vi "82_Ultrasonic_map.vi"() -> ()   [LabVIEW 2018]
uses:
  <userlib>/KNR OS 4.0 LabVIEW Toolkit/Type Definition/Resource.ctl
  <userlib>/KNR OS 3.0 LabVIEW Toolkit/Type Definition/Ultrasonic Port Number.ctl
  <userlib>/KNR OS 4.0 LabVIEW Toolkit/Type Definition/RC Servo Port.ctl
panel:
  out "Dist 1(cm)":dbl
  out "XY Graph":cluster{dbl[], dbl[]}(graph)
  in  "stop":bool
  # "500~2500"
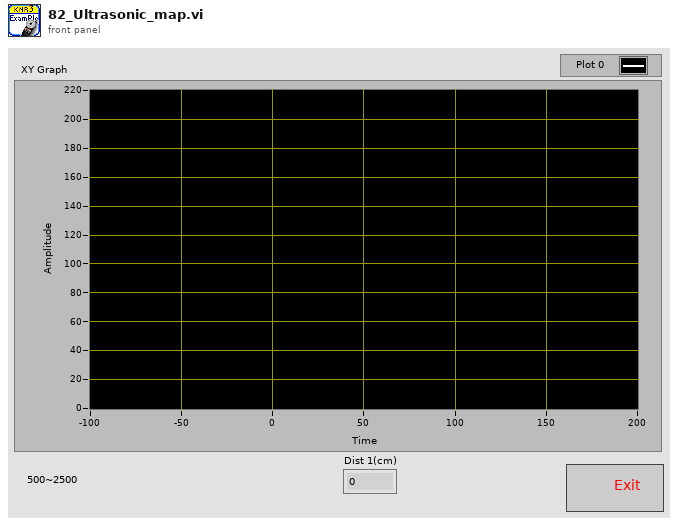
[diagram p1: front panel]
types:
  T1 = typedef "Resource.ctl" = enum16{"KNRm_DDRC", "KNRm_DDDD", "KNRm_DDDR", "KNRm_DDDC", "KNR", "KNRm_neww"}
  T2 = typedef "KNR3 Reference.ctl" = cluster{"FPGA Session":refnum<class "FPGA Interface Base.lvclass">, "Resource":T1}
  T3 = typedef "RC Servo Port.ctl" = u16
  T4 = typedef "Ultrasonic Port Number.ctl" = u16
  T5 = cluster{"Dist 1(cm)":dbl, "Dist 2(cm)":dbl, "Dist 3 (cm)":dbl, "Dist 4 (cm)":dbl}
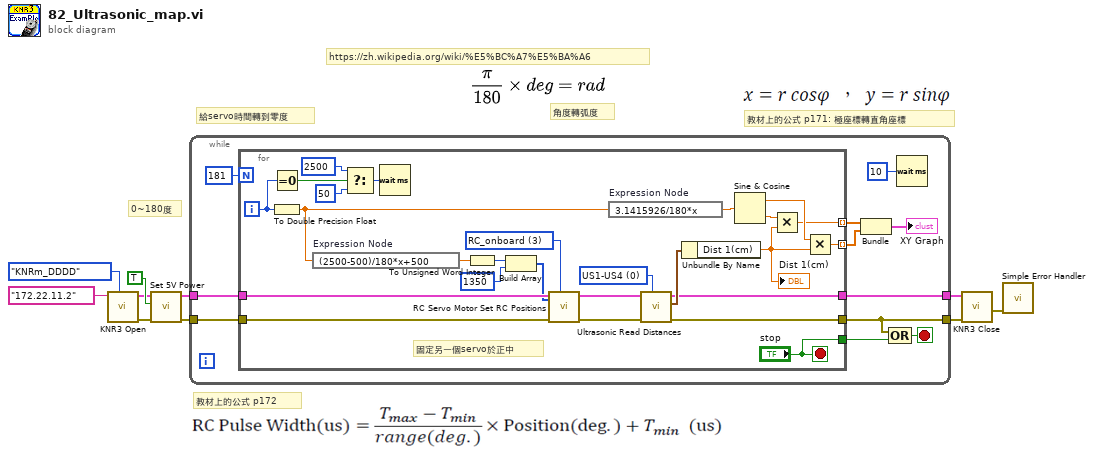
[diagram p0: block diagram]
diagram:
  # "角度轉弧度"
  # "教材上的公式 p171: 極座標轉直角座標"
  # "0~180度"
  # "給servo時間轉到零度"
  # "https://zh.wikipedia.org/wiki/%E5%BC%A7%E5%BA%A6"
  # "教材上的公式 p172"
  n1 = call <userlib>:"KNR3 Open.vi"("Resource"=Resource."KNRm_DDDD", "IP"="172.22.11.2") -> ("error out"=w8:errorcluster, "KNR out"=w9:T2)  [unwired: 8 in]
  n2 = call <userlib>:"Set 5V Power.vi"("error in (no error)"=w8, "5V Power(T)"=TRUE ("5V Power"), "KNR in"=w9) -> ("error out"=w4:errorcluster, "KNR out"=w5:T2)  [unwired: 7 in]
  n3 = while {
    tunnel: w5 -> [w21]
    tunnel: w4 -> [w20]
    tunnel: [w17] -> w2
    tunnel: [w18] -> w1
    stop <- w16 stop-if-true
    n4 = for {
      N: 181 -> [_]
      tunnel: w21 -> [w38]
      tunnel: [w30] -> w18
      tunnel: w20 -> [w37]
      tunnel: [w27] -> w17
      tunnel: [w40] -> w15 mode=indexing
      tunnel: [w39] -> w14 mode=indexing
      tunnel: ["stop"] -> w11
      i -> [w23]
      stop <- "stop" stop-if-true
      w47 = T3 3 items=["RC_onboard"=3, "RC_box"=9] ("RC Motor")
      w45 = T4 0 items=["US1-US4"=0, "US5-US8"=2] ("Port (US1-US4 for KNR)")
      # "固定另一個servo於正中"
      n5 = Equal To 0?(x=w23) -> (x = 0?=w36:bool)
      n6 = To Double Precision Float(number=w23) -> (double precision float=w26:dbl)
      n7 = expression code="(2500-500)/180*x+500"(w26) -> (w29:dbl)
      n8 = Select(t=u32 2500 ("f"), s=w36, f=u32 50 ("millisecond multiple")) -> (s? t:f=w35:u32)
      n9 = Wait (ms)(milliseconds to wait=w35) -> ()  [unwired: 1 out]
      n10 = To Unsigned Word Integer(number=w29) -> (unsigned 16bit integer=w25:u16)
      n11 = Build Array(w25, u16 1350 ("y")) -> (w28:u16[])
      n12 = call <userlib>:"RC Servo Motor Set RC Positions.vi"("Port (RC_onboard)"=w47, "error in (no error)"=w37, "RC Pulse Width (1500 uS)"=w28, "KNR in"=w38) -> ("error out"=w31:errorcluster, "KNR out"=w32:T2)  [unwired: 6 in]
      n13 = expression code="3.1415926/180*x"(w26) -> (w24:dbl)
      n14 = call <userlib>:"Ultrasonic Read Distances.vi"("Port (US1-US4 for KNR)"=w45, "error in (no error)"=w31, "KNR in"=w32) -> ("error out"=w27:errorcluster, "Ultrasonic output"=w44:T5, "KNR out"=w30:T2)  [unwired: 6 in]
      n15 = Unbundle By Name "Unbundle By Name"(w44) -> ("Dist 1(cm)"=w43:dbl)
      "Dist 1(cm)" <- w43
      n16 = Sine & Cosine(0:w24) -> (1:w41:dbl, 2:w42:dbl)
      n17 = Multiply(x=w42, y=w43) -> (x*y=w40:dbl)
      n18 = Multiply(x=w41, y=w43) -> (x*y=w39:dbl)
    }
    n19 = Bundle "Bundle"(w15, w14) -> (→"XY Graph":cluster{dbl[], dbl[]})  [unwired: 1 in]
    n20 = Compound Arithmetic op=OR(w17, w11) -> (w16:bool)
    n21 = Wait (ms)(milliseconds to wait=u32 10) -> ()  [unwired: 1 out]
  }
  n22 = call <userlib>:"KNR3 Close.vi"("error in (no error)"=w2, "KNR in"=w1) -> ("error out"=w3:errorcluster)  [unwired: 9 in]
  n23 = call <vilib>:"Simple Error Handler.vi"("error in (no error)"=w3) -> ()  [unwired: 4 in, 5 out]
